vi "String Array Delete Duplicates.vi"(1 "Array":string[](array[string])) -> (0 "Output array":string[](array[string]))   [LabVIEW 2018]
doc: "Delete duplicate items in String array."
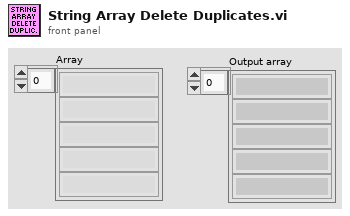
[diagram p1: front panel]
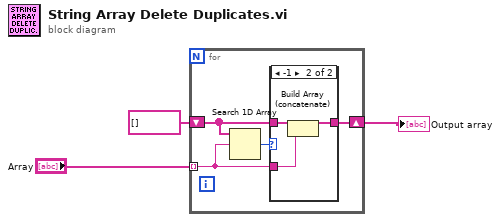
[diagram p0: block diagram]
diagram:
  n1 = for {
    tunnel: "Array" -> [w6] mode=indexing
    shift-right: [w5] -> w2
    shift-left: string[] [] -> [w4]
    n2 = Search 1D Array(1D array=w4, element=w6) -> (index of element=w7:i32)  [unwired: 1 in]
    n3 = case shown="-1" w7 {
      tunnel: w6 -> [_ w11]
      tunnel: [w8 w9] -> w5
      tunnel: w4 -> [w8 w10]
      frame Default {
      }
      frame -1 {
        n4 = Build Array (concatenate)(w10, w11) -> (w9:string[])
      }
    }
  }
  "Output array" <- w2
